vi "msc_zerowe_kw.vi"(9 "b":dbl, 10 "a":dbl, 11 "delta":dbl) -> (1 "selector":i16, 2 "x2":cdb, 3 "x1":cdb)   [LabVIEW 2020]
doc: "miejsca zerowe funkci kwadratowej"
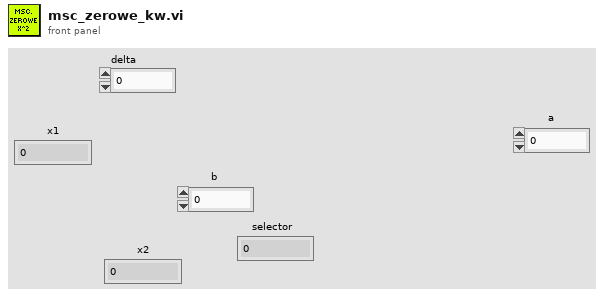
[diagram p1: front panel]
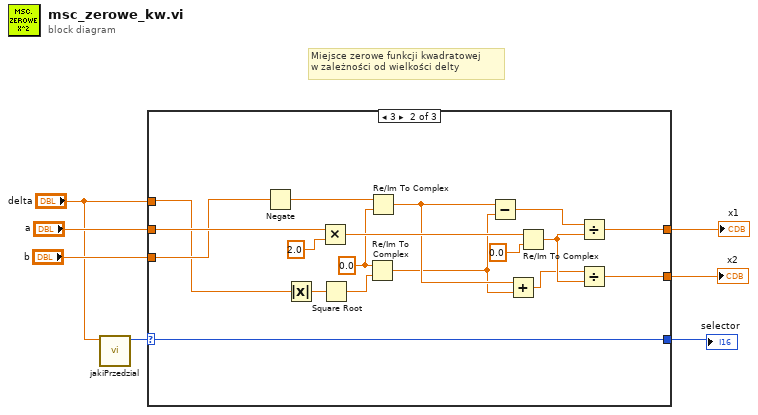
[diagram p0: block diagram]
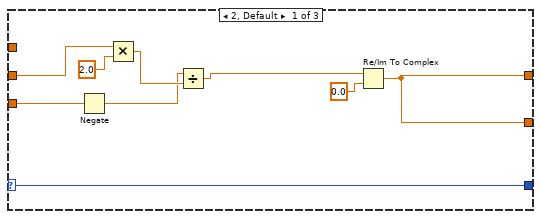
[diagram p2: hidden frame]
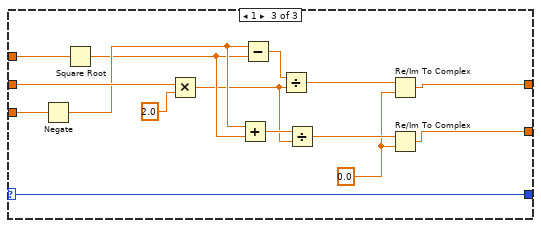
[diagram p3: hidden frame]
diagram:
  # "Miejsce zerowe funkcji kwadratowej \nw zależności od wielkości delty"
  n1 = call "jakiPrzedzial.vi"("wejscie"="delta") -> ("selector"=w1:i16)  [unwired: 10 in]
  n2 = case shown="3" w1 {
    selector: w1 -> [w8 w29 w35]
    tunnel: "delta" -> [_ w32 w49]
    tunnel: "a" -> [w16 w34 w47]
    tunnel: "b" -> [w14 w33 w45]
    tunnel: [w10 w31 w37] -> w5
    tunnel: [w10 w30 w39] -> w4
    tunnel: [w8 w29 w35] -> w3
    frame 2, Default {
      n3 = Negate(x=w14) -> (-x=w12:dbl)
      n4 = Multiply(x=w16, y=2.0) -> (x*y=w13:dbl)
      n5 = Divide(x=w12, y=w13) -> (x/y=w11:dbl)
      n6 = Re/Im To Complex(1:0.0 ("y"), 2:w11) -> (0:w10:cdb)
    }
    frame 3 {
      w21 = 0.0 ("x")
      n7 = Negate(x=w33) -> (-x=w28:dbl)
      n8 = Absolute Value(x=w32) -> (abs(x)=w17:dbl)
      n9 = Multiply(x=w34, y=2.0) -> (x*y=w25:dbl)
      n10 = Square Root(x=w17) -> (sqrt(x)=w24:dbl)
      n11 = Re/Im To Complex(1:w24, 2:w21) -> (0:w19:cdb)
      n12 = Re/Im To Complex(1:w21, 2:w28) -> (0:w20:cdb)
      n13 = Subtract(x=w20, y=w19) -> (x-y=w22:cdb)
      n14 = Add(x=w20, y=w19) -> (x+y=w18:cdb)
      n15 = Re/Im To Complex(1:0.0 ("y"), 2:w25) -> (0:w26:cdb)
      n16 = Divide(x=w22, y=w26) -> (x/y=w31:cdb)
      n17 = Divide(x=w18, y=w26) -> (x/y=w30:cdb)
    }
    frame 1 {
      w36 = 0.0 ("y")
      n18 = Negate(x=w45) -> (-x=w44:dbl)
      n19 = Square Root(x=w49) -> (sqrt(x)=w43:dbl)
      n20 = Multiply(x=w47, y=2.0) -> (x*y=w41:dbl)
      n21 = Add(x=w44, y=w43) -> (x+y=w42:dbl)
      n22 = Subtract(x=w44, y=w43) -> (x-y=w48:dbl)
      n23 = Divide(x=w48, y=w41) -> (x/y=w38:dbl)
      n24 = Divide(x=w42, y=w41) -> (x/y=w40:dbl)
      n25 = Re/Im To Complex(1:w36, 2:w38) -> (0:w37:cdb)
      n26 = Re/Im To Complex(1:w36, 2:w40) -> (0:w39:cdb)
    }
  }
  "x1" <- w5
  "x2" <- w4
  "selector" <- w3
